vi "Read Configuration File.vi"(8 "error in (no error)":errorcluster, 11 "Example Instrument in":refnum<class "Instrument.Template.lvclass">) -> (0 "error out":errorcluster, 3 "Example Instrument out":refnum<class "Instrument.Template.lvclass">)   [LabVIEW 2019, in "Instrument.Template.lvclass"]
uses:
  Instrument.Template.lvclass
  C:/Users/patrick/Documents/GitHub/Instrument-Framework/lvsrc/SMOs/Instrument/Instrument.lvclass
  SMOs/Instrument/Instrument.lvclass/Instrument.ctl
  Instrument.Template.lvclass/Instrument.Template.ctl
  SMOs/Configuration/Configuration.lvclass
  SMOs/Instrument/Instrument.lvclass
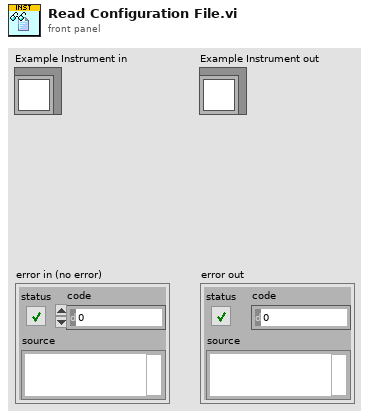
[diagram p1: front panel]
types:
  T1 = typedef "Instrument.Template.lvclass/Instrument.Template.Configuration--Cluster.ctl" = cluster{"Example Setting 1":dbl, "Example Setting 2":dbl, "Example Setting 3":string}
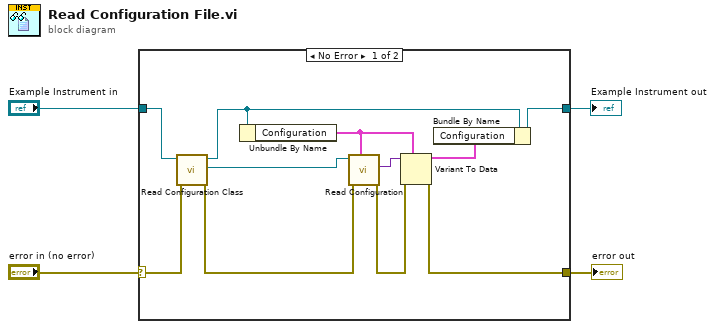
[diagram p0: block diagram]
diagram:
  n1 = case shown="No Error" "error in (no error)" {
    selector: "error in (no error)" -> [w9 w17]
    tunnel: "Example Instrument in" -> [w12 w16]
    tunnel: [w7 w16] -> w3
    tunnel: [w10 w17] -> w2
    frame No Error {
      n2 = call "Read Configuration Class.vi"("error in (no error)"=w9, "Instrument in"=w12) -> ("error out"=w13:errorcluster, "Configuration.lvclass"=w14:refnum<class "Configuration.lvclass">, "Instrument out"=w6:refnum<class "Instrument.Template.lvclass">)  [unwired: 7 in]
      n3 = Unbundle By Name(w6) -> ("Configuration"=w8:T1)
      n4 = call "Read Configuration.vi"("INI Fomatted Cluster Type"=w8, "error in (no error)"=w13, "Configuration in"=w14) -> ("error out"=w15:errorcluster, "Configuration"=w5:variant)  [unwired: 6 in, 1 out]
      n5 = Variant To Data(error in=w15, type=w8, Variant=w5) -> (data=w11:T1, error out=w10:errorcluster)
      n6 = Bundle By Name(cluster=w6, "Configuration"=w11) -> (w7:refnum<class "Instrument.Template.lvclass">)
    }
    frame Error {
    }
  }
  "Example Instrument out" <- w3
  "error out" <- w2
